vi "Parallel Index VIs.vi"(7 "Queue in":refnum<queue>, 8 "error in (no error)":errorcluster, 9 "Parallel Instances (8)":i32=8, 10 "Node Progress ref":refnum<vi>, 11 "Example Files":path[](array[path])) -> (0 "error out":errorcluster, 2 "Indexed":set{string}(c389), 3 "Node to child array":T1(array[numeric]))   [LabVIEW 2024]
uses:
  Indexer Action.ctl
  DBMap/DBMap.lvclass
  DBSet/DBSet.lvclass
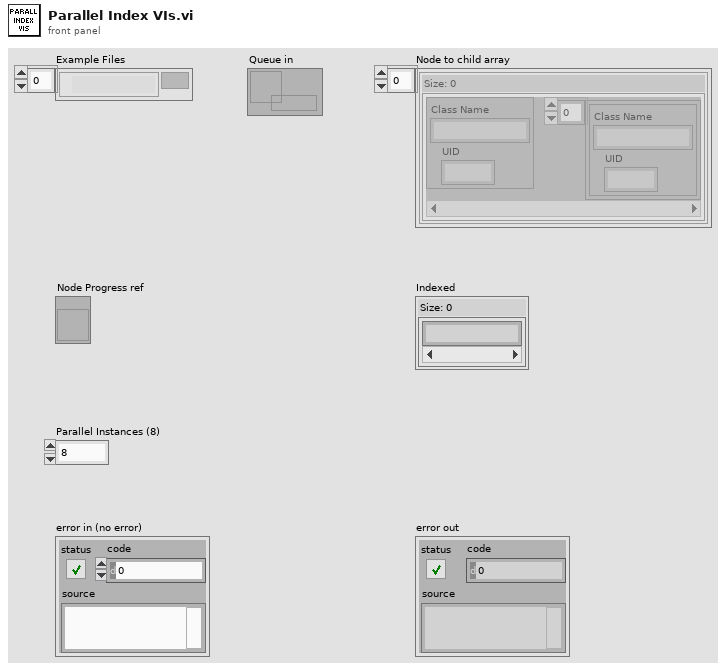
[diagram p1: front panel]
types:
  T1 = map{cluster{"Class Name":string, "UID":i32}, cluster{"Class Name":string, "UID":i32}[]}[]
  T2 = map{cluster{"Class Name":string, "UID":i32}, cluster{"Class Name":string, "UID":i32}[]}
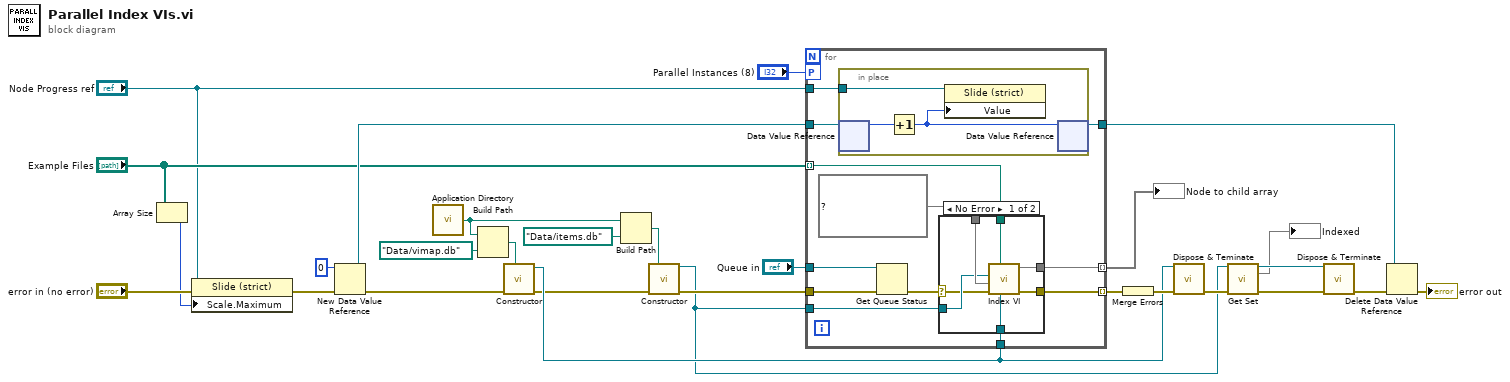
[diagram p0: block diagram]
diagram:
  n1 = Array Size(array="Example Files") -> (size(s)=w7:i32)
  n2 = property on="Property Node" class="Slide (strict)"(reference="Node Progress ref", error in="error in (no error)", "Scale.Maximum"=w7) -> (error out=w8:errorcluster)  [unwired: 1 out]
  n3 = New Data Value Reference(data value=u64 0, error in=w8) -> (data value reference=w28:refnum<data-value>, error out=w21:errorcluster)
  n4 = call <vilib>:"Application Directory.vi"() -> ("Application Directory"=w23:path)
  n5 = Build Path(base path=w23, name or relative path=path "Data/vimap.db") -> (appended path=w22:path)
  n6 = call "Constructor.vi"("SQLite DB Path"=w22, "error in (no error)"=w21) -> ("error out"=w17:errorcluster, "DBMap out"=w18:refnum<class "DBMap.lvclass">)  [unwired: 8 in]
  n7 = Build Path(base path=w23, name or relative path=path "Data/items.db") -> (appended path=w14:path)
  n8 = call "Constructor.vi"("SQLite DB Path"=w14, "error in (no error)"=w17) -> ("DBSet out"=w15:refnum<class "DBSet.lvclass">, "error out"=w16:errorcluster)  [unwired: 12 in]
  n9 = for {
    tunnel: "Example Files" -> [w40] mode=indexing
    tunnel: [w41] -> w5 mode=indexing
    tunnel: w28 -> [w39]
    tunnel: [w38] -> w27
    tunnel: w15 -> [w37]
    tunnel: w18 -> [w36]
    workers-P: "Parallel Instances (8)" -> [_]
    tunnel: w16 -> [w33]
    tunnel: [w35] -> w24 mode=indexing
    tunnel: "Queue in" -> [w34]
    tunnel: "Node Progress ref" -> [w30]
    n10 = in-place {
      in-place-border: w30 -> [w50]
      n11 = in-place-dvr #1(w39) -> (w51:u64)  [unwired: 1 out]
      n12 = Increment(x=w51) -> (x+1=w49:u64)
      n13 = property class="Slide (strict)"(reference=w50, "Value"=w49) -> ()  [unwired: 1 in, 2 out]
      n14 = in-place-dvr #1(w49) -> (w38:refnum<data-value>)  [unwired: 1 out]
    }
    n15 = Get Queue Status(queue=w34, error in (no error)=w33) -> (error out=w31:errorcluster)  [unwired: 1 in, 7 out]
    n16 = case shown="No Error" w31 {
      selector: w31 -> [w42 _]
      tunnel: set{string} {"ControlTerminal", "OverridableParameterTerminal", "ParameterTerminal", "Terminal"} ("Set") -> [w48 _]
      tunnel: [w47 _] -> w41
      tunnel: w40 -> [w46 _]
      tunnel: w37 -> [w45 _]
      tunnel: [w43 _] -> w35
      tunnel: w36 -> [w44 _]
      frame No Error {
        n17 = call "Index VI.vi"("DBMap"=w44, "VI to analyze"=w46, "error in (no error)"=w42, "Valid Terminals Set"=w48, "AtomicSet"=w45) -> ("error out"=w43:errorcluster, "Node to children"=w47:T2)  [unwired: 5 in]
      }
      frame Error {
      }
    }
  }
  "Node to child array" <- w5
  n18 = Merge Errors(w24) -> (w20:errorcluster)
  n19 = call-dynamic "Dispose & Teminate.vi"("DBMap in"=w18, "error in (no error)"=w20) -> ("error out"=w19:errorcluster)  [unwired: 12 in, 1 out]
  n20 = call "Get Set.vi"("DBSet in"=w15, "error in (no error)"=w19) -> ("DBSet out"=w11:refnum<class "DBSet.lvclass">, "Set"=→"Indexed":set{string}, "error out"=w13:errorcluster)  [unwired: 11 in]
  n21 = call-dynamic "Dispose & Terminate.vi"("DBSet in"=w11, "error in (no error)"=w13) -> ("error out"=w12:errorcluster)  [unwired: 12 in, 1 out]
  n22 = Delete Data Value Reference(data value reference=w27, error in=w12) -> (error out=→"error out":errorcluster)  [unwired: 1 out]
